vi "2D-ShapeBuilder.vi"(11 "Number of Sides":i32=3) -> (2 "Y out":dbl[](array[numeric])=[1.0, -0.4999999999999998, -0.5000000000000004, 1.0], 3 "X out":dbl[](array[numeric])=[0.0, 0.8660254037844387, -0.8660254037844384, 0.0])   [LabVIEW 2014]
doc: "André Romero - 2018\nandretec@ifsc.usp.br\n\n2D Shape Builder"
panel:
  out "XY Graph":cluster{dbl[], dbl[]}(graph)={[0.0, 0.8660254037844387, -0.8660254037844384, 0.0], [1.0, -0.4999999999999998, -0.5000000000000004, 1.0]}
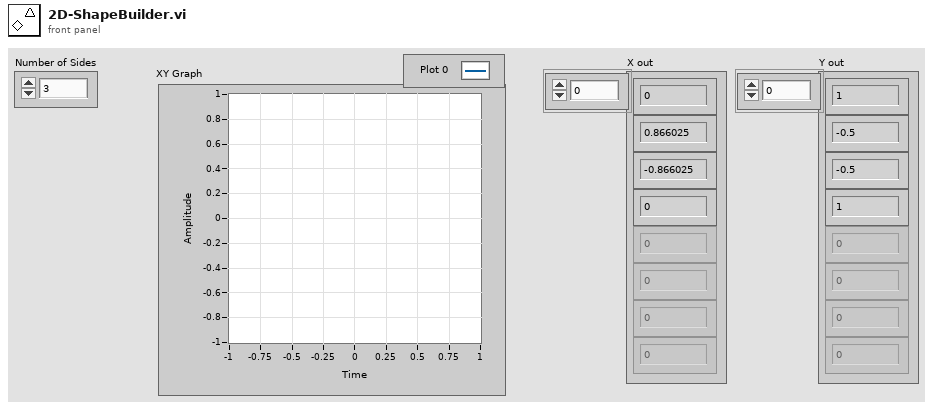
[diagram p1: front panel]
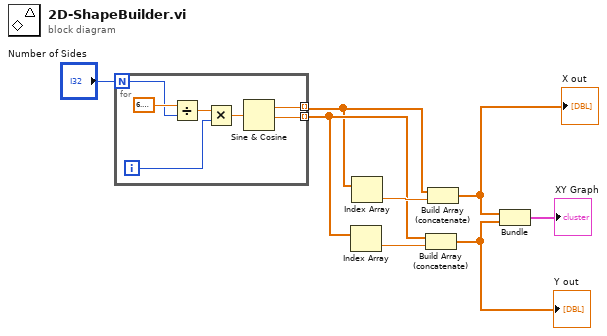
[diagram p0: block diagram]
diagram:
  n1 = for {
    N: "Number of Sides" -> [w14]
    tunnel: [w10] -> w3 mode=indexing
    tunnel: [w9] -> w4 mode=indexing
    i -> [w12]
    n2 = Divide(x=6.283185307179586, y=w14) -> (x/y=w13:dbl)
    n3 = Multiply(x=w13, y=w12) -> (x*y=w11:dbl)
    n4 = Sine & Cosine(0:w11) -> (1:w10:dbl, 2:w9:dbl)
  }
  n5 = Index Array(array=w4) -> (element=w5:dbl)  [unwired: 1 in]
  n6 = Index Array(array=w3) -> (element=w6:dbl)  [unwired: 1 in]
  n7 = Build Array (concatenate)(w4, w5) -> (w1:dbl[])
  "Y out" <- w1
  n8 = Build Array (concatenate)(w3, w6) -> (w2:dbl[])
  "X out" <- w2
  n9 = Bundle(w2, w1) -> (→"XY Graph":cluster{dbl[], dbl[]})  [unwired: 1 in]
